vi "Lock Panel.vi"(8 "error in":errorcluster, 10 "Lock Display":bool caption="Enable Shutter State (F:OFF)", 11 "EXFO in":refnum<class "EXFO.lvclass">=refnum) -> (0 "error out":errorcluster, 3 "EXFO out":refnum<class "EXFO.lvclass">)   [LabVIEW 2017]
doc: "This is a parent VI, the child VI will overwrite the functionality of this VI. \n\nThe purpose of the VI is to Tare/Zero the Power Meter. Programmatically, it must be confirmed that no input signal is injected into the system (or that the reference signal is input).\n\nAuthor: Ron Dexter\nCompany: Luminar\nModified: 5/20/2018"
uses:
  EXFO/EXFO.lvlibp/EXFO.lvclass
  LTB-1.lvclass
  EXFO/Configuration.lvlibp/Configuration.lvclass
  EXFO/EXFO.lvlibp/Methods/Read Resource.vi
  EXFO 3150/EXFO 3150.lvlib
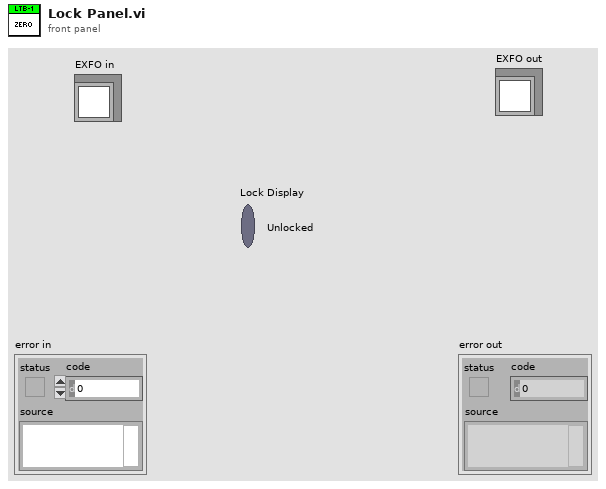
[diagram p1: front panel]
types:
  T1 = enum16{"Calibration", "PowerReading", "AttentuationReading", "Shutter"}
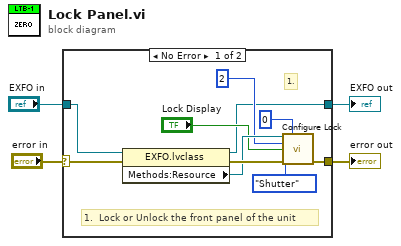
[diagram p0: block diagram]
diagram:
  n1 = case shown="No Error" "error in" {
    selector: "error in" -> [w7 w16]
    tunnel: [w12 w16] -> w4
    tunnel: "EXFO in" -> [w5 w15]
    tunnel: [w8 w15] -> w2
    frame No Error {
      # "1.  Lock or Unlock the front panel of the unit"
      # "1."
      n2 = property class="EXFO.lvclass"(reference=w5, error in=w7) -> (reference out=w8:refnum<class "EXFO.lvclass">, error out=w14:errorcluster, "Methods:Resource"=w13:refnum<visa-resource-name>)
      n3 = call "Configure Lock.vi"("VISA resource name"=w13, "Platform"=i16 0, "Module Slot Number (10)"=i16 2, "Lock Display (F:OFF)"="Lock Display", "Enum"=T1."Shutter", "error in (no error)"=w14) -> ("error out"=w12:errorcluster)  [unwired: 8 in, 1 out]
    }
    frame Error {
    }
  }
  "error out" <- w4
  "EXFO out" <- w2
